vi "Generate Simulated Data.vi"(8 "error in (no error)":T2 caption="entrée d'erreur (pas d'erreur)", 11 "Type de signal":T1) -> (0 "error out":T2 caption="sortie d'erreur", 2 "Données du graphe":waveform(dbl)[](array[waveform]))   [LabVIEW 2018, in "Acquisition.lvlib"]
doc: "Génère des exemples de waveforms en fonction du type de signal dans l'entrée Configuration du matériel."
uses:
  Acquisition.lvlib
  Signal Type.ctl
  <vilib>/Analysis/NI_AALBase.lvlib
panel:
  in  "nom du périphérique":tag="Dev1"
  out "Graphe déroulant":dynamicdata(graph)
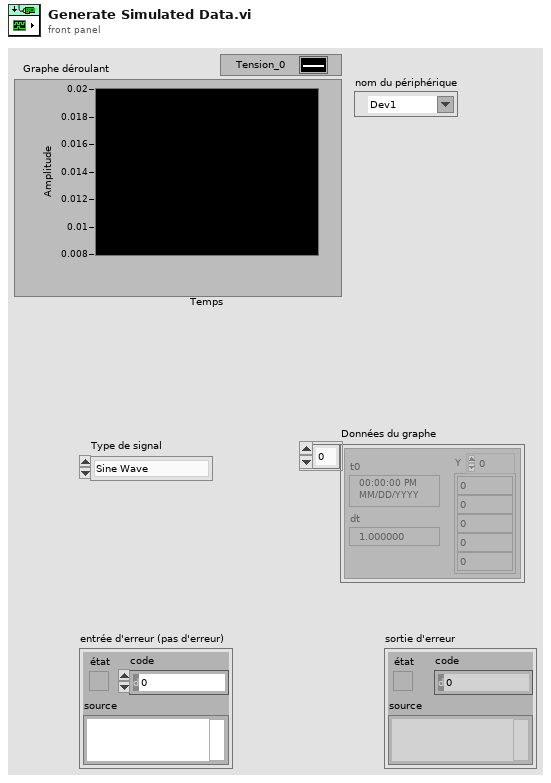
[diagram p1: front panel]
types:
  T1 = typedef "Acquisition.lvlib/Signal Type.ctl" = enum16{"Sine Wave", "Square with Noise", "Signal triangulaire", "Simulation DAQ"}
  T2 = cluster{"état":bool, "code":i32, "source":string}
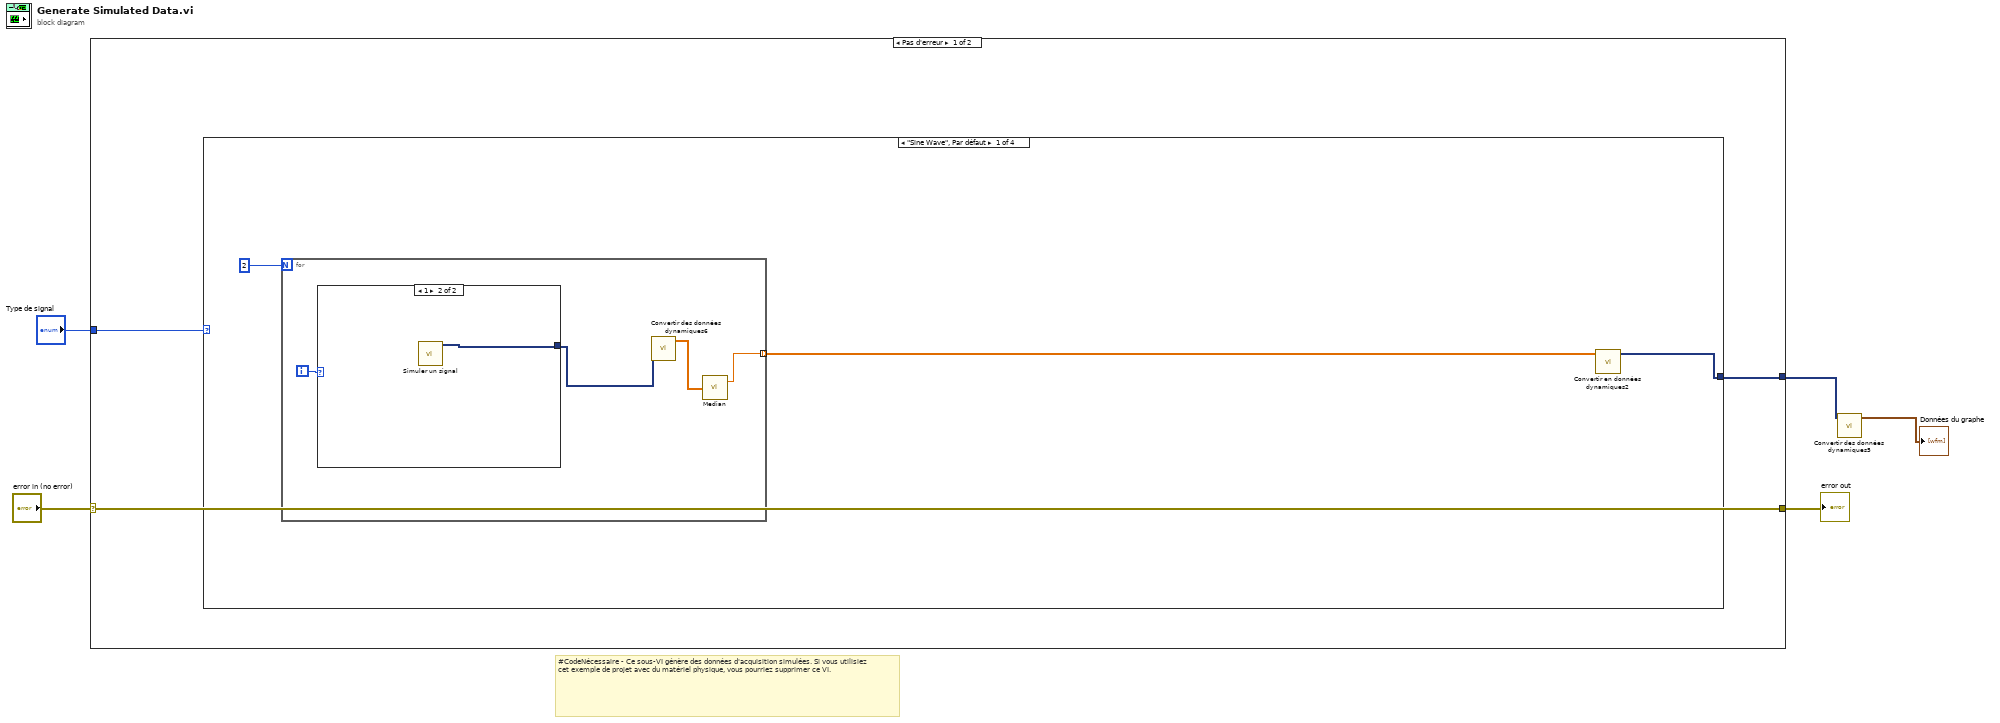
[diagram p0: block diagram]
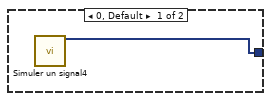
[diagram p2: hidden frame]
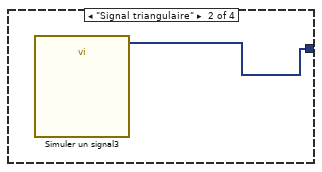
[diagram p3: hidden frame]
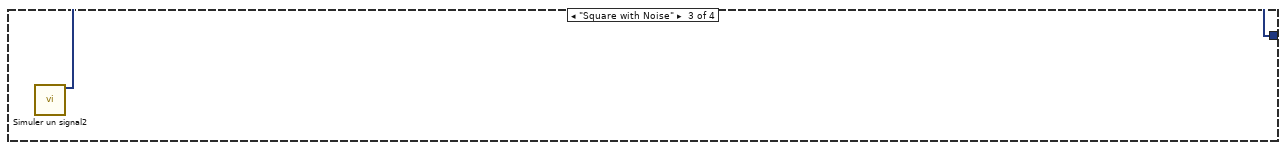
[diagram p4: hidden frame]
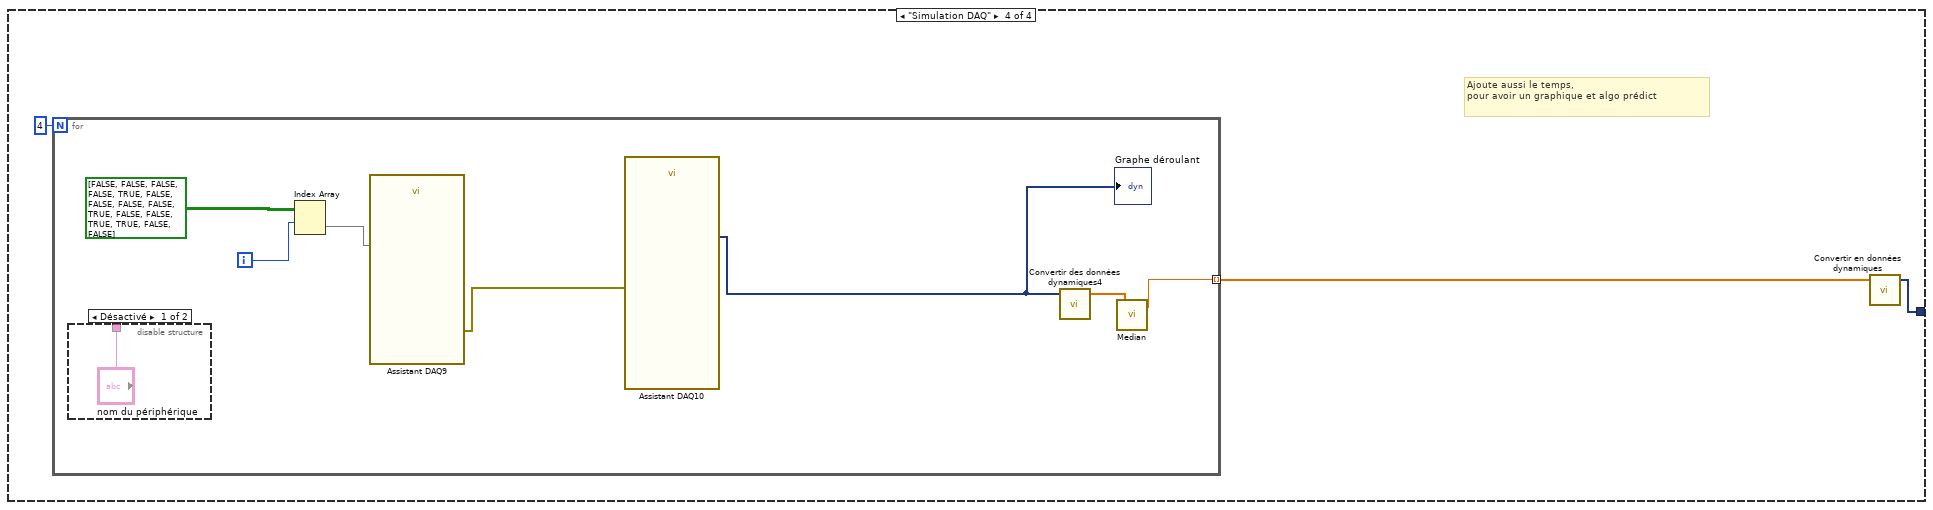
[diagram p5: hidden frame]
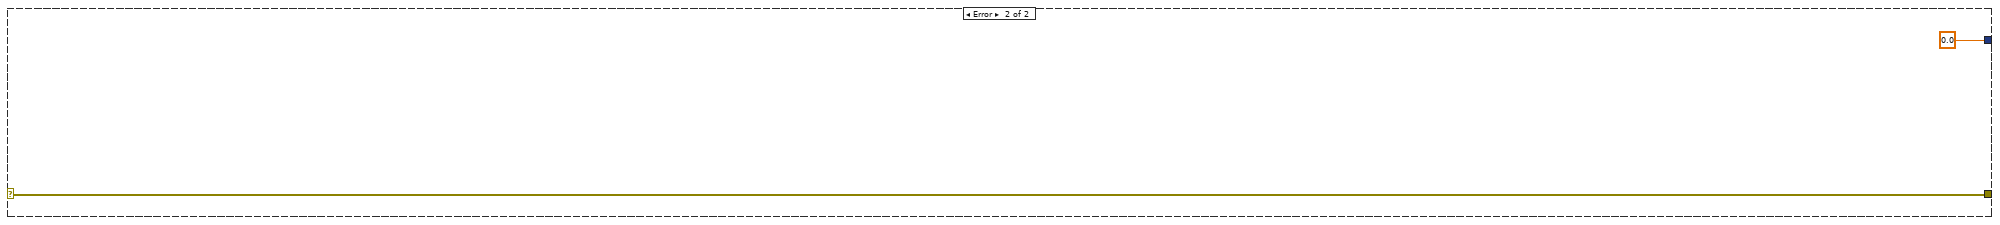
[diagram p7: hidden frame]
diagram:
  # "#CodeNécessaire - Ce sous-VI génère des données d'acquisition simulées. Si vous utilisiez cet exemple de projet avec du matériel physique, vous pourriez supprimer ce VI."
  n1 = case shown="Pas d'erreur" "error in (no error)" {
    selector: "error in (no error)" -> [w8 w32]
    tunnel: [w8 w32] -> w4
    tunnel: "Type de signal" -> [w7 _]
    tunnel: [w6 0.0] -> w1
    frame No Error {
      n2 = case shown="\"Sine Wave\", Par défaut" w7 {
        tunnel: [w10 w18 w19 w21] -> w6
        frame "Sine Wave", Default {
          n3 = for {
            N: 2 -> [_]
            tunnel: [w12] -> w9 mode=indexing
            i -> [w15]
            n4 = case shown="1" w15 {
              tunnel: [w16 w17] -> w14
              frame 0, Default {
                n5 = call "Simuler un signal4"() -> ("CC"=w16:dynamicdata)  [unwired: 14 in, 1 out]
              }
              frame 1 {
                n6 = call "Simuler un signal"() -> ("Sinus avec Bruit uniforme"=w17:dynamicdata)  [unwired: 14 in, 1 out]
              }
            }
            n7 = call "Convertir des données dynamiques6"("Dynamic Data Type"=w14) -> ("Array"=w13:dbl[])  [unwired: 3 in]
            n8 = call <vilib>:"Median.vi"("X"=w13) -> ("median"=w12:dbl)  [unwired: 1 out]
          }
          n9 = call "Convertir en données dynamiques2"("Array"=w9) -> ("Dynamic Data Type"=w10:dynamicdata)  [unwired: 3 in]
        }
        frame "Signal triangulaire" {
          n10 = call "Simuler un signal3"() -> ("Triangle"=w18:dynamicdata)  [unwired: 14 in, 1 out]
        }
        frame "Square with Noise" {
          n11 = call "Simuler un signal2"() -> ("Square with Gaussian Noise"=w19:dynamicdata)  [unwired: 14 in, 1 out]
        }
        frame "Simulation DAQ" {
          # "Ajoute aussi le temps,\npour avoir un graphique et algo prédict"
          n12 = for {
            N: 4 -> [_]
            tunnel: [w29] -> w20 mode=indexing
            i -> [w24]
            n13 = disable-structure shown="Désactivé" {
              disable-tunnel: ["nom du périphérique" _] -> _
              frame Disabled {
              }
              frame Enabled {
              }
            }
            n14 = Index Array(array=bool[][] [[FALSE, FALSE, FALSE, FALSE], [TRUE, FALSE, FALSE, FALSE], [FALSE, TRUE, FALSE, FALSE], [TRUE, TRUE, FALSE, FALSE]], index (row)=w24) -> (element=w23:bool[])  [unwired: 1 in]
            n15 = call "Assistant DAQ9"("data"=w23) -> ("error out"=w27:errorcluster)  [unwired: 17 in, 1 out]
            n16 = call "Assistant DAQ10"("error in"=w27) -> ("data"=w26:dynamicdata)  [unwired: 16 in, 2 out]
            "Graphe déroulant" <- w26
            n17 = call "Convertir des données dynamiques4"("Dynamic Data Type"=w26) -> ("Array"=w28:dbl[])  [unwired: 3 in]
            n18 = call <vilib>:"Median.vi"("X"=w28) -> ("median"=w29:dbl)  [unwired: 1 out]
          }
          n19 = call "Convertir en données dynamiques"("Array"=w20) -> ("Dynamic Data Type"=w21:dynamicdata)  [unwired: 3 in]
        }
      }
    }
    frame Error {
    }
  }
  "error out" <- w4
  n20 = call "Convertir des données dynamiques5"("Dynamic Data Type"=w1) -> ("Array of Waveform"=→"Données du graphe":waveform(dbl)[])  [unwired: 3 in]
